vi "GT Get Crd Prm.vi"(8 "error in (no error)":errorcluster caption="错误输入（无错误）", 9 "pCrdPrm":T1, 10 "crd":i16, 11 "cardNum":i16) -> (0 "error out":errorcluster caption="错误输出", 1 "pCrdPrm out":T1, 3 "function return":i16)   [LabVIEW 2014, in "gts.lvlib"]
doc: "GT_API GT_GetCrdPrm(short cardNum,short crd,TCrdPrm *pCrdPrm);"
uses:
  gts.lvlib
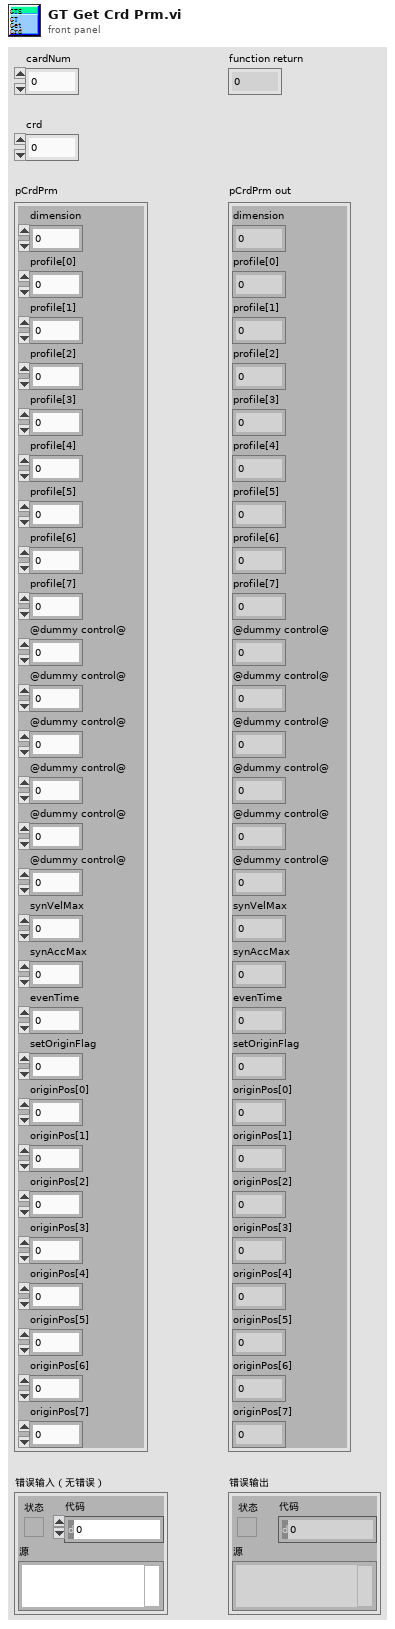
[diagram p1: front panel]
types:
  T1 = cluster{"dimension":i16, "profile[0]":i16, "profile[1]":i16, "profile[2]":i16, "profile[3]":i16, "profile[4]":i16, "profile[5]":i16, "profile[6]":i16, "profile[7]":i16, "@dummy control@":i8, "@dummy control@":i8, "@dummy control@":i8, "@dummy control@":i8, "@dummy control@":i8, "@dummy control@":i8, "synVelMax":dbl, "synAccMax":dbl, "evenTime":i16, "setOriginFlag":i16, "originPos[0]":i32, "originPos[1]":i32, "originPos[2]":i32, "originPos[3]":i32, "originPos[4]":i32, "originPos[5]":i32, "originPos[6]":i32, "originPos[7]":i32}
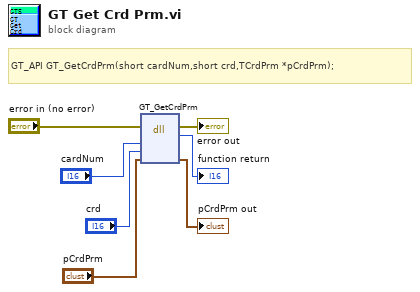
[diagram p0: block diagram]
diagram:
  # "GT_API GT_GetCrdPrm(short cardNum,short crd,TCrdPrm *pCrdPrm);"
  n1 = dll-call lib="PTH2habs D固高科技资料GTS控制卡GTS卡18年上半年资料dllVC32bit\nmulti_cardgts.*" fn="GT_GetCrdPrm"(error in="error in (no error)", "cardNum"="cardNum", "crd"="crd", "pCrdPrm"="pCrdPrm") -> (error out=→"error out":errorcluster, →"function return":i16, "pCrdPrm"=→"pCrdPrm out":T1)  [unwired: 4 in, 1 out]
